vi "runtime io test.vi"() -> ()   [LabVIEW 2013, in "Profibus Module tests.lvlib"]
uses:
  Profibus Module tests.lvlib
  <vilib>/NI/Tag Bus/dictionary/data dictionary.lvclass
  <vilib>/NI/Tag Bus/table/data table.lvlib
  <vilib>/NI/Tag Bus/table/data polymorphs/write one/write Double.vi
  <vilib>/NI/Tag Bus/table/data polymorphs/read one/read Double.vi
  execution/Profibus Module runtime.lvclass
  channel/Profibus channel.lvclass
panel:
  out "inputs changed?":bool
  out "no error":errorcluster
  # "This is expected to remain false until you write code for input"
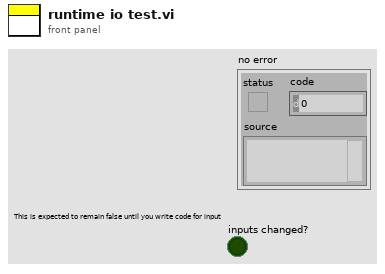
[diagram p1: front panel]
types:
  T1 = typedef "tag bus.lvlib/tag descriptor.lvclass/Data Type.ctl" = enum16{"Double", "Single", "I64", "I32", "I16", "I8", "U64", "U32", "U16", "U8", "Boolean", "String", "Array of Double", "Array of Single", "Array of I64", "Array of I32", "Array of I16", "Array of I8", "Array of U64", "Array of U32", "Array of U16", "Array of U8", "Array of Boolean", "Array of String"}
  T2 = typedef "TBM channel.lvclass/data tables.ctl" = cluster{"input data":T3, "processing parameter":T3, "processing result":T3, "output data":T3}
  T3 = typedef "tag bus.lvlib/dictionary table pair.ctl" = cluster{"data dictionary":refnum<class "data dictionary.lvclass">, "data table":T4}
  T4 = typedef "tag bus.lvlib/data table.lvlib/data table.ctl" = cluster{"Double":dbl[], "Single":sgl[], "I64":i64[], "I32":i32[], "I16":i16[], "I8":i8[], "U64":u64[], "U32":u32[], "U16":u16[], "U8":u8[], "Boolean":bool[], "String":string[], "Array of Double":cluster{"DBL Array":dbl[]}[], "Array of Single":cluster{"SGL Array":sgl[]}[], "Array of I64":cluster{"I64 Array":i64[]}[], "Array of I32":cluster{"I32 Array":i32[]}[], "Array of I16":cluster{"I16 Array":i16[]}[], "Array of I8":cluster{"I8 Array":i8[]}[], "Array of U64":cluster{"U64 Array":u64[]}[], "Array of U32":cluster{"U32 Array":u32[]}[], "Array of U16":cluster{"U16 Array":u16[]}[], "Array of U8":cluster{"U8 Array":u8[]}[], "Array of Boolean":cluster{"Boolean Array":bool[]}[], "Array of String":cluster{"String Array":string[]}[]}
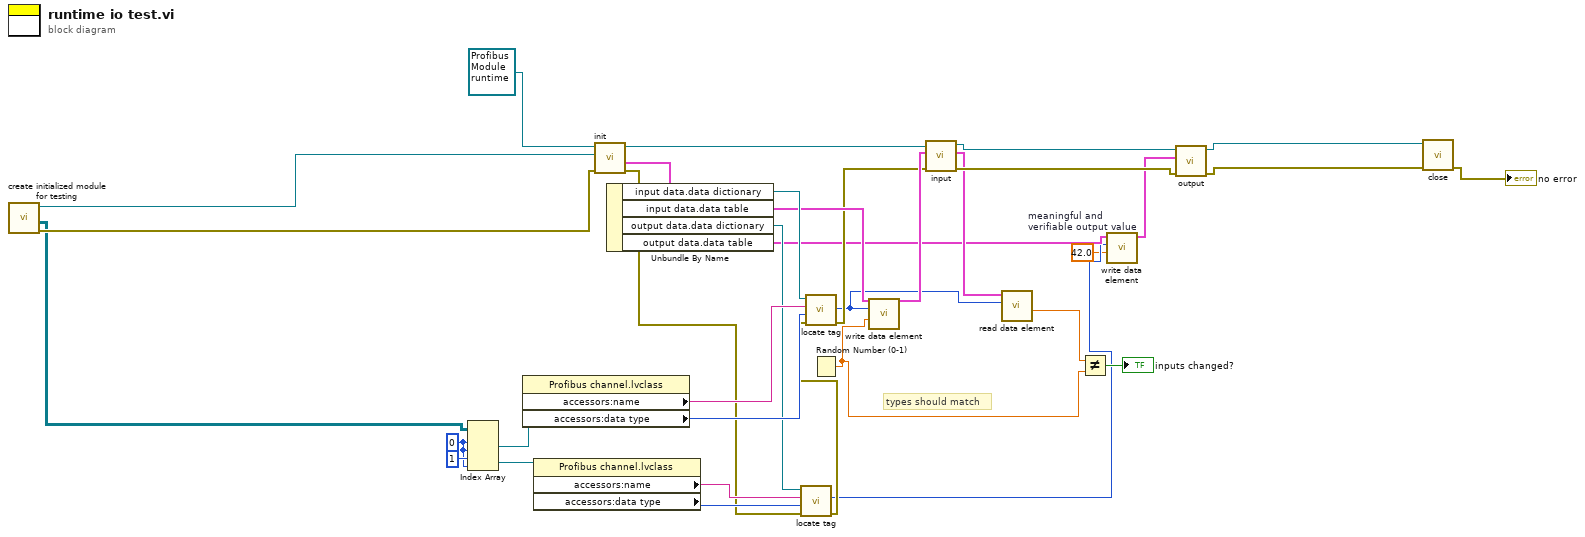
[diagram p0: block diagram]
diagram:
  w1 = 0 ("index (row)")
  w7 = 42.0  # meaningful and verifiable output value
  # "types should match"
  n1 = call "create initialized module for testing.vi"() -> ("error out"=w4:errorcluster, "2d channels"=w3:refnum<class "Profibus channel.lvclass">[][], "Profibus Module configuration out"=w5:refnum<class "Profibus Module configuration.lvclass">)  [unwired: 6 in, 3 out]
  n2 = Index Array(array=w3, index (row) #1=w1, index (col) #1=w1, index (row) #2=1 ("index (row)"), index (col) #2=w1) -> (element #1=w27:refnum<class "Profibus channel.lvclass">, element #2=w16:refnum<class "Profibus channel.lvclass">)
  n3 = property class="Profibus channel.lvclass"(reference=w27) -> ("accessors:name"=w25:string, "accessors:data type"=w26:T1)  [unwired: 1 in, 2 out]
  n4 = property class="Profibus channel.lvclass"(reference=w16) -> ("accessors:name"=w14:string, "accessors:data type"=w13:T1)  [unwired: 1 in, 2 out]
  n5 = call-dynamic "init.vi"("error in"=w4, "TBM module configuration in"=w5, "Profibus Module runtime in"=refnum<class "Profibus Module runtime.lvclass"> refnum ("tag bus configurable plugin module")) -> ("error out"=w12:errorcluster, "data allocations"=w29:T2, "Profibus Module runtime out"=w30:refnum<class "Profibus Module runtime.lvclass">)  [unwired: 5 in, 1 out]
  n6 = Unbundle By Name(w29) -> ("input data.data dictionary"=w28:refnum<class "data dictionary.lvclass">, "input data.data table"=w24:T4, "output data.data dictionary"=w15:refnum<class "data dictionary.lvclass">, "output data.data table"=w10:T4)
  n7 = call <vilib>:"locate tag.vi"("error in"=w12, "data type"=w13, "name"=w14, "data dictionary in"=w15) -> ("error out"=w11:errorcluster, "index"=w8:i32)  [unwired: 5 in, 1 out]
  n8 = call <vilib>:"locate tag.vi"("error in"=w11, "data type"=w26, "name"=w25, "data dictionary in"=w28) -> ("error out"=w22:errorcluster, "index"=w20:i32)  [unwired: 5 in, 1 out]
  n9 = Random Number (0-1)() -> (number: 0 to 1=w19:dbl)
  n10 = call-poly <vilib>:"write data element.vi"("value"=w19, "index"=w20, "data table in"=w24) -> ("data table out"=w23:T4)  [unwired: 8 in]
  n11 = call-dynamic "input.vi"("error in"=w22, "data table in"=w23, "Profibus Module runtime in"=w30) -> ("error out"=w31:errorcluster, "data table out"=w21:T4, "Profibus Module runtime out"=w32:refnum<class "Profibus Module runtime.lvclass">)  [unwired: 6 in]
  n12 = call-poly <vilib>:"read data element.vi"("index"=w20, "data table in"=w21) -> ("value"=w18:dbl)  [unwired: 8 in, 1 out]
  n13 = Not Equal?(x=w18, y=w19) -> (x != y?=→"inputs changed?":bool)
  n14 = call-poly <vilib>:"write data element.vi"("value"=w7, "index"=w8, "data table in"=w10) -> ("data table out"=w9:T4)  [unwired: 8 in]
  n15 = call-dynamic "output.vi"("error in"=w31, "data table in"=w9, "Profibus Module runtime in"=w32) -> ("error out"=w33:errorcluster, "Profibus Module runtime out"=w34:refnum<class "Profibus Module runtime.lvclass">)  [unwired: 6 in, 1 out]
  n16 = call-dynamic "close.vi"("error in"=w33, "Profibus Module runtime in"=w34) -> ("error out"=→"no error":errorcluster)  [unwired: 9 in]
